vi "Get controls on tabs.vi"(8 "error in":errorcluster, 11 "Pages":refnum<vi>[](array[refnum])) -> (0 "error out":errorcluster, 2 "Cntrl Ref":refnum<vi>[](array[refnum]), 3 "Cntrl Labels":string[](array[string]))   [LabVIEW 2014]
doc: "This VI returns a Reference to All The Contols that Exist on a Tab Control as well as the Label for each of those Controls."
panel:
  in  "GetClassIDTab":enum32{"Page 1", "Page 2"}(tab)
  in  "Controls on Page[]":refnum<vi>[](array[refnum])
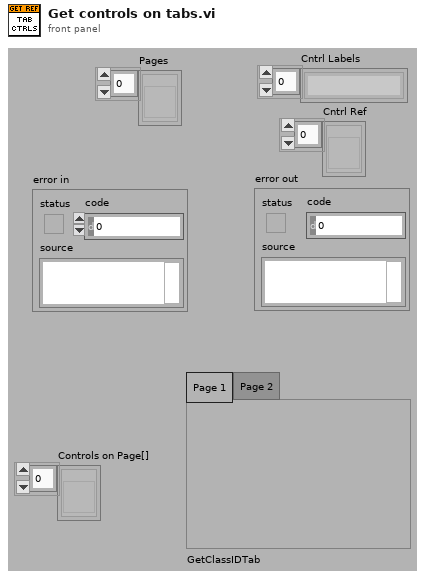
[diagram p1: front panel]
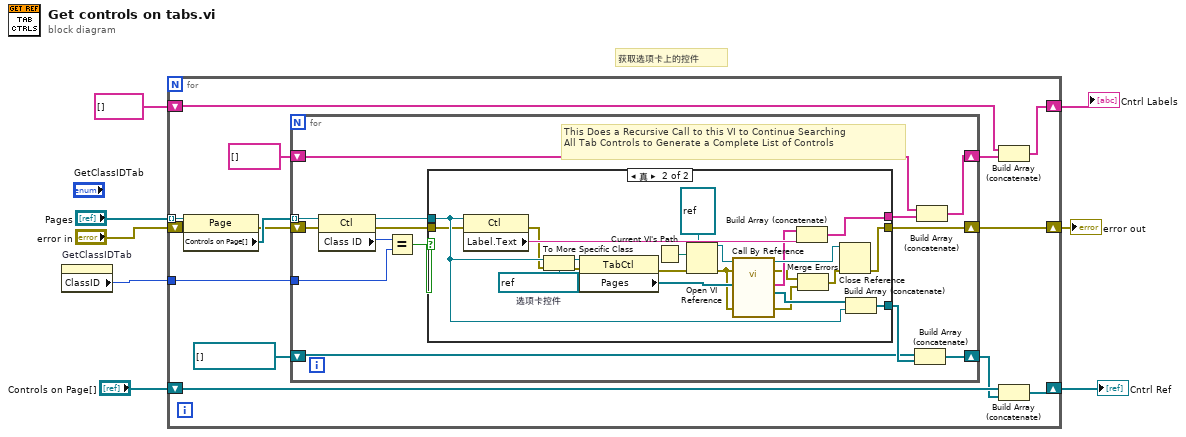
[diagram p0: block diagram]
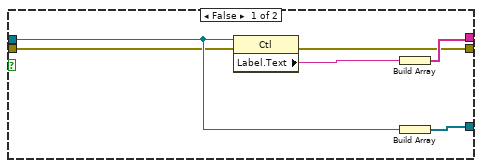
[diagram p2: hidden frame]
diagram:
  # "获取选项卡上的控件"
  n1 = property on="GetClassIDTab" class="TabCtl (严格)"() -> ("ClassID"=w1:u32)  [unwired: 2 in, 2 out]
  n2 = for {
    tunnel: "Pages" -> [w22] mode=indexing
    shift-right: [w21] -> w5
    shift-left: string[] [] -> [w20]
    shift-right: [w19] -> w4
    shift-left: "Controls on Page[]" -> [w18]
    shift-right: [w10] -> w2
    shift-left: "error in" -> [w11]
    tunnel: w1 -> [w9]
    n3 = property class="Page"(reference=w22, error in=w11) -> (error out=w16:errorcluster, "Controls on Page[]"=w17:refnum<vi>[])  [unwired: 1 out]
    n4 = for {
      tunnel: w17 -> [w36] mode=indexing
      shift-right: [w28] -> w14
      shift-left: string[] [] -> [w30]
      shift-right: [w33] -> w15
      shift-left: refnum<vi>[] [] -> [w31]
      shift-right: [w24] -> w10
      shift-left: w16 -> [w26]
      tunnel: w9 -> [w23]
      # "This Does a Recursive Call to this VI to Continue Searching\nAll Tab Controls to Generate a Complete List of Controls"
      n5 = property class="Ctl"(reference=w36, error in=w26) -> (reference out=w27:refnum<vi>, error out=w25:errorcluster, "Class ID"=w35:u32)
      n6 = Equal?(x=w35, y=w23) -> (x = y?=w34:bool)
      n7 = case shown="真" w34 {
        tunnel: w27 -> [w41 w61]
        tunnel: [w42 w63] -> w32
        tunnel: [w39 w59] -> w29
        tunnel: w25 -> [w38 w58]
        tunnel: [w37 w47] -> w24
        frame False {
          n8 = property class="Ctl"(reference=w41, error in=w38) -> (error out=w37:errorcluster, "Label.Text"=w40:string)  [unwired: 1 out]
          n9 = Build Array(w40) -> (w39:string[])
          n10 = Build Array(w41) -> (w42:refnum<vi>[])
        }
        frame True {
          w64 = refnum<vi> refnum  # 选项卡控件
          n11 = property class="Ctl"(reference=w61, error in=w58) -> (error out=w49:errorcluster, "Label.Text"=w60:string)  [unwired: 1 out]
          n12 = To More Specific Class(target class=w64, reference=w61, error in=w49) -> (specific class reference=w62:refnum<vi>, error out=w50:errorcluster)
          n13 = property class="TabCtl"(reference=w62, error in=w50) -> (error out=w48:errorcluster, "Pages"=w53:refnum<vi>[])  [unwired: 1 out]
          n14 = Current VI's Path() -> (path=w55:path)
          n15 = Open VI Reference(type specifier VI Refnum (for type only)=refnum<vi> refnum, vi path=w55, error in (no error)=w48) -> (vi reference=w57:refnum<vi>, error out=w46:errorcluster)  [unwired: 3 in]
          n16 = call-by-ref "?"(reference=w57, error in=w46, "error in"=w46, "Pages"=w53) -> (reference out=w56:refnum<vi>, error out=w45:errorcluster, 0:"error out"=w43:errorcluster, "Cntrl Ref"=w51:refnum<vi>[], "Cntrl Labels"=w52:string[])  [unwired: 7 in]
          n17 = Build Array (concatenate)(w52, w60) -> (w59:string[])
          n18 = Merge Errors(w45, w43) -> (w44:errorcluster)
          n19 = Close Reference(reference=w56, error in (no error)=w44) -> (error out=w47:errorcluster)
          n20 = Build Array (concatenate)(w51, w61) -> (w63:refnum<vi>[])
        }
      }
      n21 = Build Array (concatenate)(w31, w32) -> (w33:refnum<vi>[])
      n22 = Build Array (concatenate)(w30, w29) -> (w28:string[])
    }
    n23 = Build Array (concatenate)(w20, w14) -> (w21:string[])
    n24 = Build Array (concatenate)(w18, w15) -> (w19:refnum<vi>[])
  }
  "Cntrl Labels" <- w5
  "Cntrl Ref" <- w4
  "error out" <- w2
